vi "Create Global MetaData Channel - Single Channel - Enumerated List.vi"(0 "Instrument Addon Refnum In":T1=18446744073709551615 format="%.0x", 1 "Name":string, 2 "Settings":T2, 3 "Error In":errorcluster) -> (7 "Instrument Addon Refnum Out":T1=18446744073709551615 format="%.0x", 8 "Channel Refnum":T1=18446744073709551615 format="%.0x", 10 "Error Out":errorcluster)   [LabVIEW 2018, in "Instrument Addon Scripting API.lvlib"]
doc: "Creates a Global MetaData Channel under the referenced Instrument Addon CD."
uses:
  Instrument Addon Scripting API.lvlib
  <vilib>/NI Veristand/Custom Device API/Custom Device Item Ref.ctl
  TypeDefs/Single Channel Enumerated List Settings.ctl
  Addon/Addon Shared/Types/MetaData Parameters.ctl
  Addon/Addon Shared/Types/Protocol Data Type.ctl
  Addon/Addon Shared/Types/Metadata Channel Type.ctl
  Addon/Addon Shared/Types/Type Cast Type.ctl
  Addon/Addon Shared/Types/Endian.ctl
  TypeDefs/Channel Properties.ctl
  TypeDefs/MetaData Channel Type.ctl
  Addon/Addon Shared/Instrument Addon Shared.lvlib
  <vilib>/NI Veristand/Custom Device API/Custom Device API.lvlib
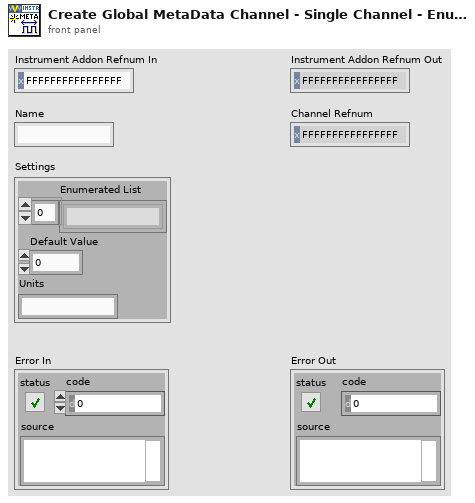
[diagram p1: front panel]
types:
  T1 = typedef "Custom Device API.lvlib/Custom Device Item Ref.ctl" = u64
  T2 = typedef "Instrument Addon Scripting API.lvlib/Single Channel Enumerated List Settings.ctl" = cluster{"Enumerated List":string[], "Default Value":dbl, "Units":string}
  T3 = typedef "MetaData Channel Type.ctl" = enum16{"MetaData", "Global MetaData"}
  T4 = typedef "Channel Properties.ctl" = cluster{"Default Value":dbl, "Units":string}
  T5 = typedef "Instrument Addon Shared.lvlib/Metadata Channel Type.ctl" = enum16{"Enumerated List", "Format", "Type Cast"}
  T6 = typedef "Instrument Addon Shared.lvlib/Protocol Data Type.ctl" = enum16{"Single Channel", "Array"}
  T7 = typedef "Instrument Addon Shared.lvlib/MetaData Parameters.ctl" = cluster{"Data Type":T6, "Channel Type":T5, "List":string[], "Format String":string, "Type":T8, "Delimiter":string, "Endian":T9}
  T8 = typedef "Instrument Addon Shared.lvlib/Type Cast Type.ctl" = enum16{"DBL", "SGL", "U64", "U32", "U16", "U8", "I64", "I32", "I16", "I8"}
  T9 = typedef "Instrument Addon Shared.lvlib/Endian.ctl" = enum16{"Native", "Little", "Big"}
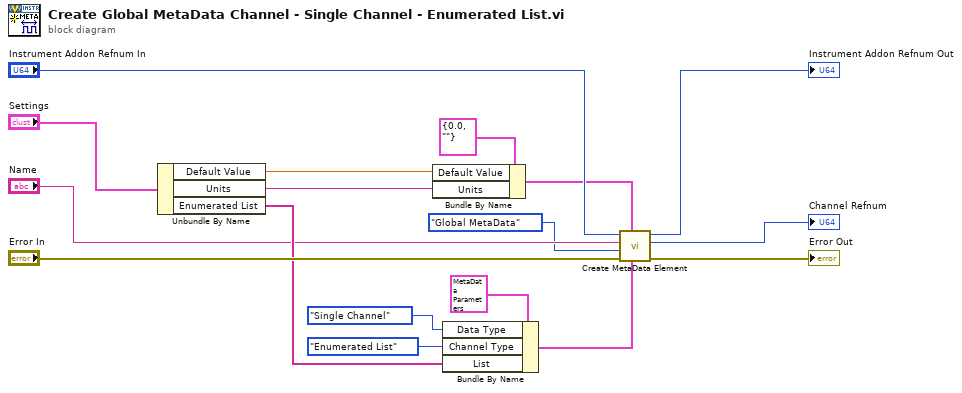
[diagram p0: block diagram]
diagram:
  n1 = Unbundle By Name("Settings") -> ("Default Value"=w8:dbl, "Units"=w7:string, "Enumerated List"=w11:string[])
  n2 = Bundle By Name(cluster=T4 {"Default Value"=0.0, "Units"=""}, "Default Value"=w8, "Units"=w7) -> (w5:T4)
  n3 = Bundle By Name(cluster=T7 {"Data Type"=enum."Single Channel", "Channel Type"=enum."Format", "List"=[], "Format String"="%.3g", "Type"=enum."SGL", "Delimiter"="", "Endian"=enum."Native"} ("MetaData Parameters"), "Data Type"=Protocol_Data_Type."Single Channel", "Channel Type"=Metadata_Channel_Type."Enumerated List", "List"=w11) -> (w10:T7)
  n4 = call "Create MetaData Element.vi"("MetaData Parameters"=w10, "Channel Properties"=w5, "error in (no error)"="Error In", "Type"=MetaData_Channel_Type."Global MetaData", "Name"="Name", "Refnum In"="Instrument Addon Refnum In") -> ("error out"=→"Error Out":errorcluster, "Channel Refnum"=→"Channel Refnum":T1, "Refnum Out"=→"Instrument Addon Refnum Out":T1)  [unwired: 3 in]
